vi "Set Temperature.vi"(8 "error in (no error)":errorcluster, 11 "Cooler in":refnum<class "Cooler.lvclass">) -> (0 "error out":errorcluster, 3 "Cooler out":refnum<class "Cooler.lvclass">)   [LabVIEW 2018, in "Cooler.lvclass"]
doc: "Este VI configura a temperatura do CCD."
uses:
  Cooler.lvclass
  Cooler.lvclass/Cooler.ctl
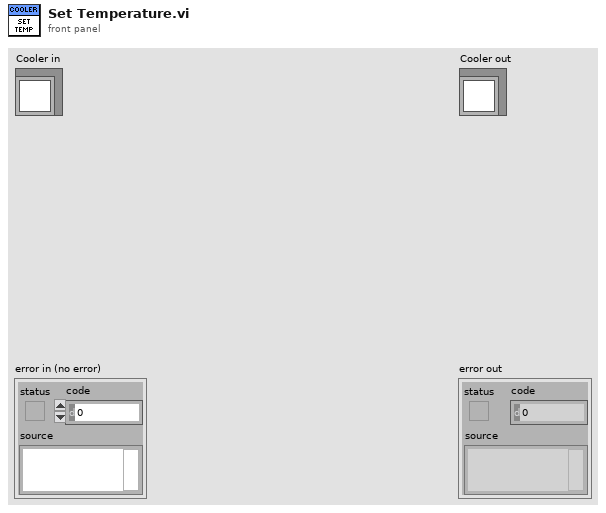
[diagram p1: front panel]
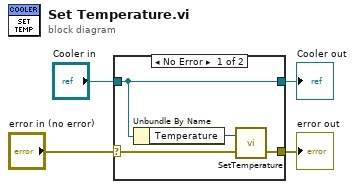
[diagram p0: block diagram]
diagram:
  n1 = case shown="No Error" "error in (no error)" {
    selector: "error in (no error)" -> [w8 w10]
    tunnel: [w7 w10] -> w1
    tunnel: [w6 w9] -> w2
    tunnel: "Cooler in" -> [w6 w9]
    frame No Error {
      n2 = Unbundle By Name(w6) -> ("Temperature"=w5:i8)
      n3 = call <userlib>:"SetTemperature.vi"("error in (no error)"=w8, "temperature"=w5) -> ("error out"=w7:errorcluster)  [unwired: 1 out]
    }
    frame Error {
    }
  }
  "error out" <- w1
  "Cooler out" <- w2
